vi "Set TEC Temps.vi"(8 "error in":errorcluster, 11 "cPAS in":refnum<class "cPAS.lvclass">) -> (0 "error out":errorcluster, 3 "cPAS out":refnum<class "cPAS.lvclass">)   [LabVIEW 2015, in "cPAS.lvclass"]
uses:
  cPAS.lvclass
  cPAS.lvclass/cPAS.ctl
  <vilib>/DAQmx/write.llb/DAQmx Write (Analog 1D DBL NChan 1Samp).vi
  <vilib>/DAQmx/miscellaneous.llb/DAQmx Fill In Error Info.vi
  Reusable/General/Temperature/Temperature.lvlib
  Reusable/Instrument/Instrument.lvclass
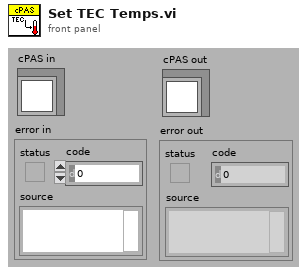
[diagram p1: front panel]
types:
  T1 = cluster{"Cell 1":sgl, "Cell 2":sgl, "Cell 3":sgl, "Cell 4":sgl, "Cell 5":sgl}
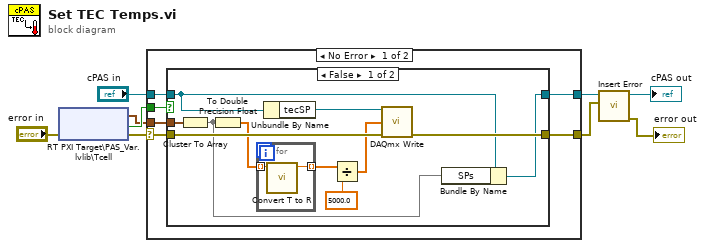
[diagram p0: block diagram]
diagram:
  n1 = shared-variable "RT PXI Target\\PAS_Var.lvlib\\Tcell"(error in="error in") -> (w8:T1, error out=w5:errorcluster, w9:bool)  [unwired: 1 in]
  n2 = case shown="No Error" w5 {
    selector: w5 -> [w10 w31]
    tunnel: w9 -> [w15 _]
    tunnel: w8 -> [w14 _]
    tunnel: "cPAS in" -> [w13 w30]
    tunnel: [w12 w30] -> w4
    tunnel: [w11 w31] -> w3
    frame No Error {
      n3 = case shown="False" w15 {
        tunnel: w14 -> [w25 _]
        tunnel: w13 -> [w18 w29]
        tunnel: [w16 w29] -> w12
        tunnel: [w23 _] -> w11
        tunnel: w10 -> [w24 _]
        frame False {
          n4 = Cluster To Array(cluster=w25) -> (array=w17:sgl[])
          n5 = To Double Precision Float(number=w17) -> (double precision float=w21:dbl[])
          n6 = for {
            tunnel: w21 -> [w28] mode=indexing
            tunnel: [w27] -> w20 mode=indexing
            n7 = call "Convert T to R.vi"("T"=w28) -> ("R"=w27:dbl)  [unwired: 10 in]
          }
          n8 = Unbundle By Name(w18) -> ("tecSP"=w26:refnum<k21>)
          n9 = Divide(x=w20, y=5000.0) -> (x/y=w19:dbl[])
          n10 = call-poly <vilib>:"DAQmx Write.vi"("task/channels in"=w26, "data"=w19, "error in"=w24) -> ("error out"=w23:errorcluster)  [unwired: 10 in, 2 out]
          n11 = Bundle By Name(cluster=w18, "SPs"=w17) -> (w16:refnum<class "cPAS.lvclass">)
        }
        frame True {
        }
      }
    }
    frame Error {
    }
  }
  n12 = call "Insert Error.vi"("err"=w3, "Instrument in"=w4) -> ("error out"=→"error out":errorcluster, "Instrument out"=→"cPAS out":refnum<class "cPAS.lvclass">)  [unwired: 7 in, 1 out]
